vi "Set URL.vi"(8 "Error In":errorcluster, 10 "URL":string, 11 "WebView in":refnum<class "WebView.lvclass">) -> (0 "Error Out":errorcluster, 3 "WebView out":refnum<class "WebView.lvclass">)   [LabVIEW 2024, in "WebView.lvclass"]
uses:
  WebView.lvclass
  WebView.lvclass/WebView.ctl
  <vilib>/sklein/WebView2/Libs/Microsoft.Web.WebView2.Core.dll
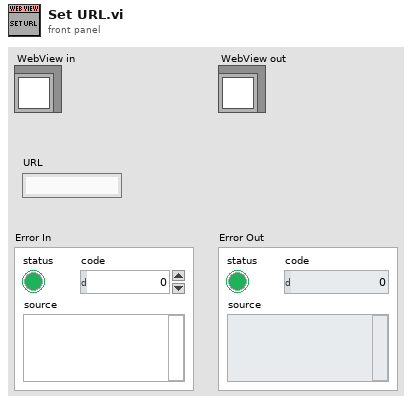
[diagram p1: front panel]
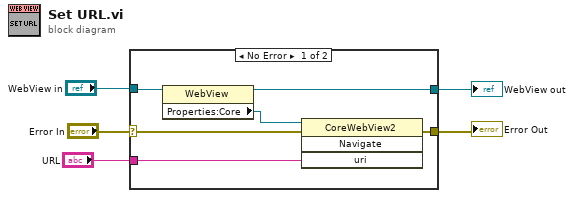
[diagram p0: block diagram]
diagram:
  n1 = case shown="No Error" "Error In" {
    selector: "Error In" -> [w7 w13]
    tunnel: [w6 w13] -> w4
    tunnel: [w10 w12] -> w2
    tunnel: "WebView in" -> [w11 w12]
    tunnel: "URL" -> [w8 _]
    frame No Error {
      n2 = property class="WebView"(reference=w11) -> (reference out=w10:refnum<class "WebView.lvclass">, "Properties:Core"=w9:refnum<k24>)  [unwired: 1 in, 1 out]
      n3 = invoke class="CoreWebView2" method="Navigate"(reference=w9, error in=w7, "uri"=w8) -> (error out=w6:errorcluster)  [unwired: 1 in, 3 out]
    }
    frame Error {
    }
  }
  "Error Out" <- w4
  "WebView out" <- w2
